vi "MSScript_Format_UpdRFChFunc.vi"(9 "ValueArray":string[](array[string]), 10 "TagArray":string[](array[string]), 11 "MSScript.lvclass":refnum<class "MSScript.lvclass">) -> (0 "ValueErrorArray":bool[](array[boolean]), 1 "TagErrorArray":bool[](array[boolean]), 2 "ParamErrorArray":bool[](array[boolean]), 3 "Data":variant, 4 "#ofParamError":bool)   [LabVIEW 2018, in "MSScript.lvclass"]
uses:
  MSScript.lvclass
  Ctl/MSEditorParam updRFChFunc.ctl
  MSScript_Transform_UInt.vi
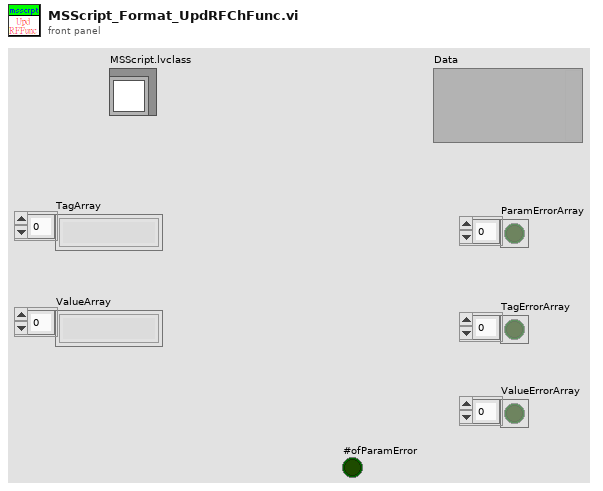
[diagram p1: front panel]
types:
  T1 = typedef "MSEditorParam updRFChFunc.ctl" = cluster{"ch1":u8, "ch2":u8, "ch3":u8}
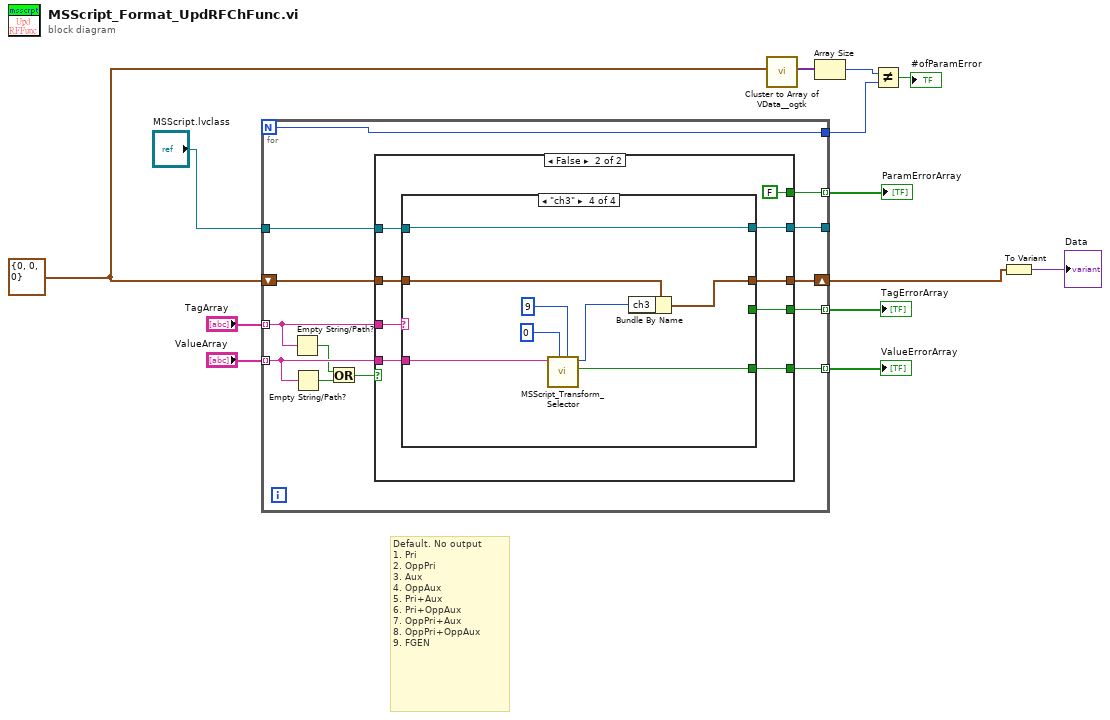
[diagram p0: block diagram]
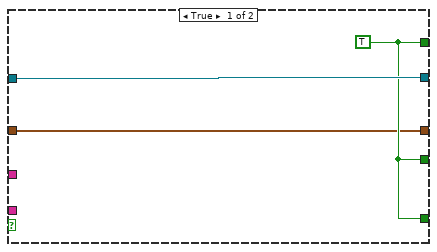
[diagram p2: hidden frame]
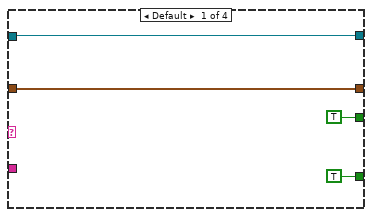
[diagram p3: hidden frame]
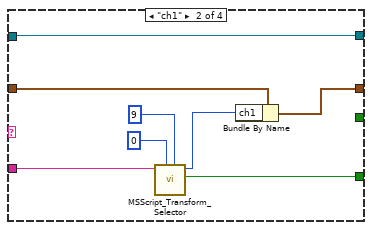
[diagram p4: hidden frame]
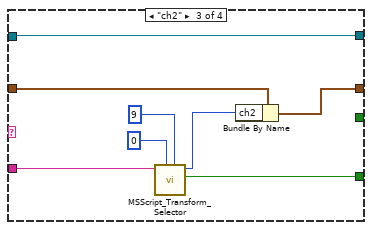
[diagram p5: hidden frame]
diagram:
  w1 = T1 {"ch1"=0, "ch2"=0, "ch3"=0} ("ParamValueType")
  # "Default. No output\n1. Pri\n2. OppPri\n3. Aux\n4. OppAux\n5. Pri+Aux\n6. Pri+OppAux\n7. OppPri+Aux\n8. OppPri+OppAux\n9. FGEN"
  n1 = for {
    N -> [w14]
    tunnel: "TagArray" -> [w22] mode=indexing
    tunnel: "ValueArray" -> [w21] mode=indexing
    tunnel: [w26] -> w11 mode=indexing
    tunnel: "MSScript.lvclass" -> [w25]
    tunnel: [w24] -> w10 mode=indexing
    tunnel: [w23] -> _
    tunnel: [w17] -> w9 mode=indexing
    shift-right: [w15] -> w3
    shift-left: w1 -> [w16]
    tunnel: [w14] -> w4
    n2 = Empty String/Path?(string/path=w22) -> (empty?=w19:bool)
    n3 = Empty String/Path?(string/path=w21) -> (empty?=w20:bool)
    n4 = Or(x=w19, y=w20) -> (x .or. y?=w18:bool)
    n5 = case shown="False" w18 {
      tunnel: [w28 w31] -> w26
      tunnel: w25 -> [w29 w34]
      tunnel: [w28 w30] -> w24
      tunnel: [w29 w33] -> w23
      tunnel: w22 -> [_ w36]
      tunnel: w21 -> [_ w37]
      tunnel: [w28 FALSE] -> w17
      tunnel: w16 -> [w27 w35]
      tunnel: [w27 w32] -> w15
      frame True {
        w28 = TRUE
      }
      frame False {
        n6 = case shown="\"ch3\"" w36 {
          tunnel: [TRUE _ _ _] -> w31
          tunnel: w37 -> [_ w49 w57 w65]
          tunnel: [TRUE ("Value Error?") w50 w58 w66] -> w30
          tunnel: [w40 w46 w54 w62] -> w33
          tunnel: [w39 w48 w56 w64] -> w32
          tunnel: w35 -> [w39 w47 w55 w63]
          tunnel: w34 -> [w40 w46 w54 w62]
          frame Default {
          }
          frame "ch1" {
            n7 = call-poly "MSScript_Transform_Selector.vi"("upper limit"=u64 9, "lower limit"=u64 0 ("upper limit"), "string in"=w49) -> ("Value Error?"=w50:bool, "Value Output"=w43:u64)  [unwired: 6 in, 1 out]
            n8 = Bundle By Name(cluster=w47, "ch1"=w43) -> (w48:T1)
          }
          frame "ch2" {
            n9 = call-poly "MSScript_Transform_Selector.vi"("upper limit"=u64 9, "lower limit"=u64 0 ("upper limit"), "string in"=w57) -> ("Value Error?"=w58:bool, "Value Output"=w51:u64)  [unwired: 6 in, 1 out]
            n10 = Bundle By Name(cluster=w55, "ch2"=w51) -> (w56:T1)
          }
          frame "ch3" {
            n11 = call-poly "MSScript_Transform_Selector.vi"("upper limit"=u64 9, "lower limit"=u64 0 ("upper limit"), "string in"=w65) -> ("Value Error?"=w66:bool, "Value Output"=w59:u64)  [unwired: 6 in, 1 out]
            n12 = Bundle By Name(cluster=w63, "ch3"=w59) -> (w64:T1)
          }
        }
      }
    }
  }
  "TagErrorArray" <- w11
  "ValueErrorArray" <- w10
  "ParamErrorArray" <- w9
  n13 = call <userlib>:"Cluster to Array of VData__ogtk.vi"("Cluster"=w1) -> ("Array of VData"=w7:variant[])  [unwired: 9 in, 1 out]
  n14 = Array Size(array=w7) -> (size(s)=w6:i32)
  n15 = Not Equal?(x=w6, y=w4) -> (x != y?=→"#ofParamError":bool)
  n16 = To Variant(anything=w3) -> (Variant=→"Data":variant)
